vi "PH_BeamlineInformation.PC _Beamline Elements.vi"(0 "i ref in":refnum<vi>, 2 "serviceName":string, 3 "State":i16, 4 "not linked?":bool, 5 "error in (no error)":errorcluster) -> (14 "i ref out":refnum<vi>, 19 "error out":errorcluster)   [LabVIEW 2014, in "PH_BeamlineInformation.lvlib"]
doc: "This VI writes the state of the beamline elements to own attributes and the GUI elements."
uses:
  PH_BeamlineInformation.lvlib
  PH_Basics/PH_Common/PH_Common.lvlib
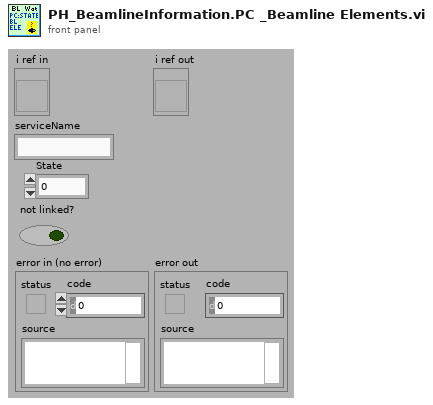
[diagram p1: front panel]
types:
  T1 = typedef "PH_BeamlineInformation.lvlib/PH_BeamlineInformation.i attribute.ctl" = cluster{"BL GUI Elements of Services":cluster{"Service Name":string, "GUI Elements":refnum<vi>[], "Status":i32}[], "Powermeters":T2, "Efficiency":T3, "Heads":T4[]}
  T2 = typedef "PH_BeamlineInformation.lvlib/PH_BeamlineInformation.Powermeter.ctl" = cluster{"ns FE":cluster{"GUI Ref":refnum<vi>, "Value":dbl}, "fs FE":cluster{"GUI Ref":refnum<vi>, "Value":dbl}, "PA":cluster{"GUI Ref":refnum<vi>, "Value":dbl}, "MA":cluster{"GUI Ref":refnum<vi>, "Value":dbl}, "Z6 green":cluster{"GUI Ref":refnum<vi>, "Value":dbl}, "Z6 IR":cluster{"GUI Ref":refnum<vi>, "Value":dbl}, "Z6 COS":cluster{"GUI Ref":refnum<vi>, "Value":dbl}}
  T3 = typedef "PH_BeamlineInformation.lvlib/PH_BeamlineInformation.Efficiency.ctl" = cluster{"PA Gain":cluster{"GUI Ref":refnum<vi>, "Value":dbl}, "MA Gain":cluster{"GUI Ref":refnum<vi>, "Value":dbl}, "Z6 green Conversion":cluster{"GUI Ref":refnum<vi>, "Value":dbl}, "Z6 Comp Losses":cluster{"GUI Ref":refnum<vi>, "Value":dbl}}
  T4 = typedef "PH_BeamlineInformation.lvlib/PH_BeamlineInformation.Head.ctl" = cluster{"PowerUnit":T5, "in use":cluster{"Value":bool, "GUI Ref":refnum<vi>, "linked":bool}, "voltage":cluster{"Value":dbl, "GUI Ref":refnum<vi>, "linked":bool}}
  T5 = typedef "PH_PP_Common.lvlib/PH_PP_Common.PUs.ctl" = enum16{"no Info", "PA-19mm-1", "PA-19mm-2", "PA-45mm-PILC", "PA-45mm-MAIN", "MA-PU-1", "MA-PU-2", "MA-PU-3", "MA-PU-4", "MA-PU-5", "MA-PU-6", "MA-FR", "MA-PILC", "PA-45mm-DP"}
  T6 = cluster{"Service Name":string, "GUI Elements":refnum<vi>[], "Status":i32}[]
  T7 = cluster{"Service Name":string, "GUI Elements":refnum<vi>[], "Status":i32}
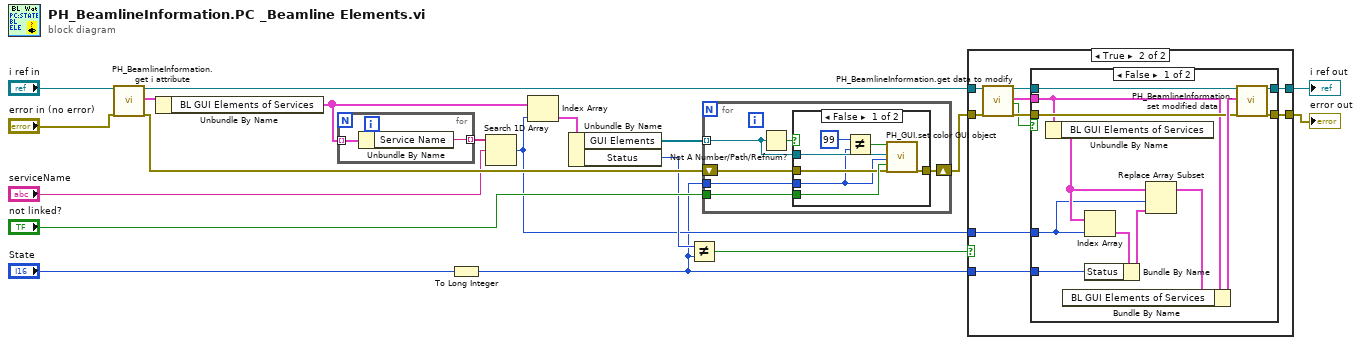
[diagram p0: block diagram]
diagram:
  n1 = call "PH_BeamlineInformation.get i attribute.vi"("i ref in"="i ref in", "error in (no error)"="error in (no error)") -> ("i ref out"=w9:refnum<vi>, "i attribute"=w19:T1, "error out"=w15:errorcluster)  [unwired: 15 in]
  n2 = Unbundle By Name(w19) -> ("BL GUI Elements of Services"=w13:T6)
  n3 = for {
    tunnel: w13 -> [w21] mode=indexing
    tunnel: [w20] -> w14 mode=indexing
    n4 = Unbundle By Name(w21) -> ("Service Name"=w20:string)
  }
  n5 = To Long Integer(number="State") -> (32bit integer=w2:i32)
  n6 = Search 1D Array(1D array=w14, element="serviceName") -> (index of element=w4:i32)  [unwired: 1 in]
  n7 = Index Array(array=w13, index=w4) -> (element=w12:T7)
  n8 = Unbundle By Name(w12) -> ("GUI Elements"=w11:refnum<vi>[], "Status"=w5:i32)
  n9 = Not Equal?(x=w5, y=w2) -> (x != y?=w1:bool)
  n10 = for {
    shift-right: [w27] -> w10
    shift-left: w15 -> [w26]
    tunnel: w2 -> [w24]
    tunnel: "not linked?" -> [w23]
    tunnel: w11 -> [w22] mode=indexing
    n11 = Not A Number/Path/Refnum?(number/path/refnum=w22) -> (NaN/Path/Refnum?=w25:bool)
    n12 = case shown="False" w25 {
      tunnel: w22 -> [w32 _]
      tunnel: [w34 w35] -> w27
      tunnel: w26 -> [w31 w35]
      tunnel: w24 -> [w28 _]
      tunnel: w23 -> [w33 _]
      frame False {
        n13 = Not Equal?(x=99, y=w28) -> (x != y?=w29:bool)
        n14 = call "PH_GUI.set color GUI object.vi"("Visible? (true)"=w29, "GUI object Ref"=w32, "State"=w28, "Blinking? (false)"=w33, "error in (no error)"=w31) -> ("error out"=w34:errorcluster)  [unwired: 14 in]
      }
      frame True {
      }
    }
  }
  n15 = case shown="True" w1 {
    tunnel: w2 -> [_ w43]
    tunnel: [w37 w40] -> w8
    tunnel: [w36 w39] -> w7
    tunnel: w9 -> [w37 w42]
    tunnel: w10 -> [w36 w41]
    tunnel: w4 -> [_ w38]
    frame False {
    }
    frame True {
      n16 = call "PH_BeamlineInformation.get data to modify.vi"("i ref in"=w42, "error in (no error)"=w41) -> ("i ref out"=w47:refnum<vi>, "i attribute"=w44:T1, "timed out"=w45:bool, "error out"=w46:errorcluster)  [unwired: 14 in]
      n17 = case shown="False" w45 {
        tunnel: [w59 w61] -> w40
        tunnel: w47 -> [w58 w61]
        tunnel: w46 -> [w55 w60]
        tunnel: [w57 w60] -> w39
        tunnel: w44 -> [w54 _]
        tunnel: w43 -> [w48 _]
        tunnel: w38 -> [w51 _]
        frame False {
          n18 = Unbundle By Name(w54) -> ("BL GUI Elements of Services"=w52:T6)
          n19 = Index Array(array=w52, index=w51) -> (element=w50:T7)
          n20 = Bundle By Name(cluster=w50, "Status"=w48) -> (w49:T7)
          n21 = Replace Array Subset(array=w52, new element=w49, index=w51) -> (w53:T6)
          n22 = Bundle By Name(cluster=w54, "BL GUI Elements of Services"=w53) -> (w56:T1)
          n23 = call "PH_BeamlineInformation.set modified data.vi"("i ref in"=w58, "i attribute"=w56, "error in (no error)"=w55) -> ("i ref out"=w59:refnum<vi>, "error out"=w57:errorcluster)  [unwired: 15 in]
        }
        frame True {
        }
      }
    }
  }
  "error out" <- w7
  "i ref out" <- w8
